vi "ProjectFile Dialog.vi"(0 "Path":path, 1 "error in":errorcluster, 6 "button label":string="Open") -> (14 "New Path":path, 15 "error out":errorcluster)   [LabVIEW 2019]
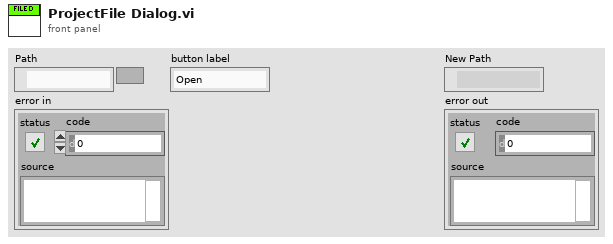
[diagram p1: front panel]
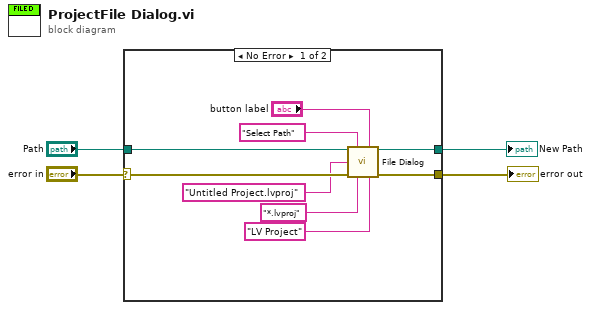
[diagram p0: block diagram]
diagram:
  n1 = case shown="No Error" "error in" {
    selector: "error in" -> [w10 w14]
    tunnel: "Path" -> [w13 _]
    tunnel: [w12 _] -> w3
    tunnel: [w11 w14] -> w2
    frame No Error {
      n2 = call "File Dialog"("start path"=w13, "prompt"="Select Path", "button label"="button label", "default name"="Untitled Project.lvproj", "error in"=w10, "pattern (all files)"="*.lvproj", "pattern label"="LV Project") -> ("selected path"=w12:path, "error out"=w11:errorcluster)  [unwired: 5 in, 2 out]
    }
    frame Error {
    }
  }
  "New Path" <- w3
  "error out" <- w2
